vi "Create VariantMsg.vi"(8 "error in (no error)":errorcluster, 10 "Message Data":variant, 11 "Message Name":string) -> (0 "error out":errorcluster, 3 "VariantMsg Out":refnum<class "VariantMsg.lvclass">)   [LabVIEW 2013, in "LapDog.Messaging.v3.NativeTypes.lvlib" / "VariantMsg.lvclass"]
doc: "Returns a VariantMsg object with the given name.\n\nThis method executes regardless of the error in state."
uses:
  VariantMsg.lvclass
  LapDog.Messaging/Message/Message.lvclass
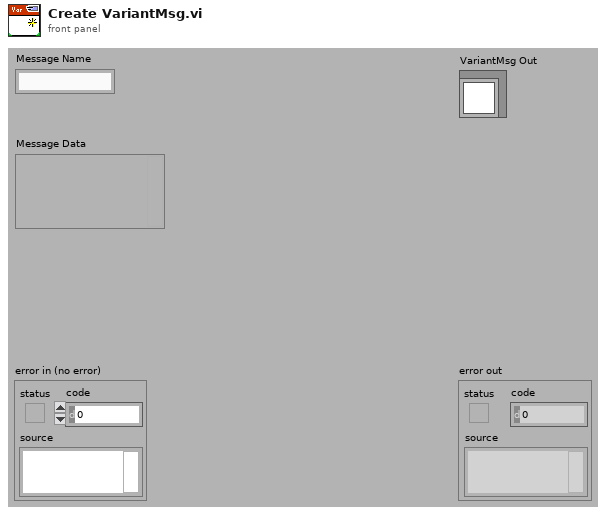
[diagram p1: front panel]
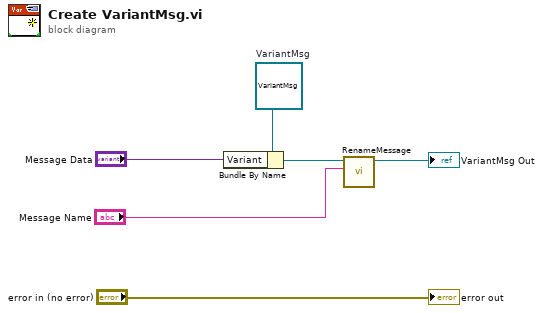
[diagram p0: block diagram]
diagram:
  w1 = refnum<class "VariantMsg.lvclass"> refnum  # VariantMsg
  n1 = Bundle By Name(cluster=w1, "Variant"="Message Data") -> (w4:refnum<class "VariantMsg.lvclass">)
  n2 = call "RenameMessage.vi"("Message Name"="Message Name", "Message in"=w4) -> ("Message out"=→"VariantMsg Out":refnum<class "VariantMsg.lvclass">)  [unwired: 8 in, 1 out]
  "error out" <- "error in (no error)"
